vi "CreateErrorString.vi"(9 "Error In":errorcluster) -> (1 "Error Out":errorcluster, 2 "Error String":string)   [LabVIEW 2016]
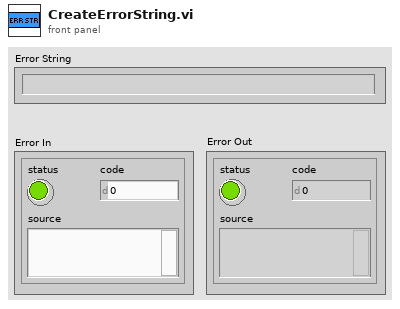
[diagram p1: front panel]
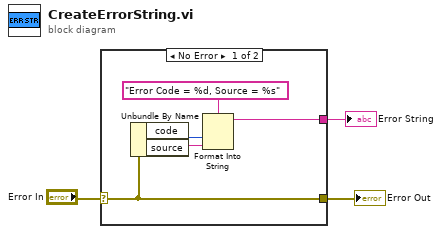
[diagram p0: block diagram]
diagram:
  n1 = case shown="No Error" "Error In" {
    selector: "Error In" -> [w4 w9]
    tunnel: [w8 _] -> w3
    tunnel: [w4 w9] -> w1
    frame No Error {
      n2 = Unbundle By Name(w4) -> ("code"=w6:i32, "source"=w7:string)
      n3 = Format Into String(format string="Error Code = %d, Source = %s", w6, w7) -> (resulting string=w8:string)  [unwired: 2 in, 1 out]
    }
    frame Error {
    }
  }
  "Error String" <- w3
  "Error Out" <- w1
